vi "mean_2D.vi"(3 "transpose":bool, 4 "filter":enum16{"none", "invalids", "zero"}(ring), 5 "2D array":dbl[][](array[numeric])) -> (0 "errors":i32[](array[numeric]), 1 "counts":i32[](array[numeric]), 2 "means":dbl[](array[numeric]))   [LabVIEW 2020]
uses:
  <vilib>/Analysis/baseanly.llb/Mean (DBL).vi
  <vilib>/Analysis/NI_AALBase.lvlib
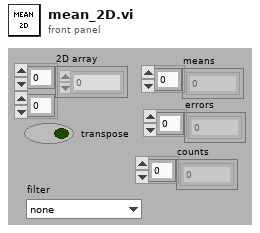
[diagram p1: front panel]
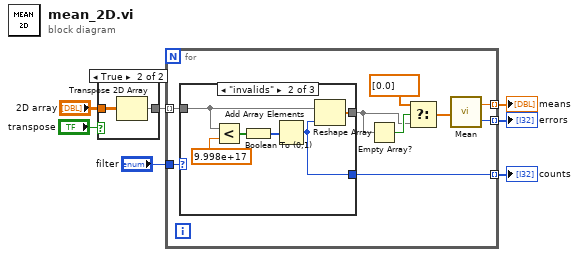
[diagram p0: block diagram]
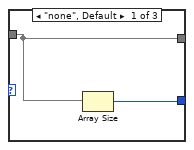
[diagram p3: hidden frame]
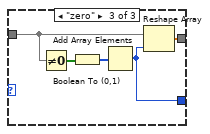
[diagram p4: hidden frame]
diagram:
  n1 = case shown="True" "transpose" {
    tunnel: "2D array" -> [w8 w10]
    tunnel: [w8 w9] -> w6
    frame False {
    }
    frame True {
      n2 = Transpose 2D Array(2D array=w10) -> (transposed array=w9:dbl[][])
    }
  }
  n3 = for {
    tunnel: w6 -> [w17] mode=indexing
    tunnel: [w19] -> w4 mode=indexing
    tunnel: [w18] -> w3 mode=indexing
    tunnel: [w16] -> w2 mode=indexing
    tunnel: "filter" -> [w15]
    n4 = case shown="\"invalids\"" w15 {
      tunnel: w17 -> [w21 w24 w28]
      tunnel: [w21 w23 w31] -> w12
      tunnel: [w20 w22 w30] -> w16
      frame "none", Default {
        n5 = Array Size(array=w21) -> (size(s)=w20:i32)
      }
      frame "invalids" {
        n6 = Less?(x=w24, y=9.998e+17) -> (x < y?=w26:bool[])
        n7 = Boolean To (0,1)(Boolean=w26) -> (0, 1=w25:i16[])
        n8 = Add Array Elements(numeric array=w25) -> (sum=w22:i16)
        n9 = Reshape Array(w24, w22) -> (w23:dbl[])
      }
      frame "zero" {
        n10 = Not Equal To 0?(x=w28) -> (x != 0?=w29:bool[])
        n11 = Boolean To (0,1)(Boolean=w29) -> (0, 1=w32:i16[])
        n12 = Add Array Elements(numeric array=w32) -> (sum=w30:i16)
        n13 = Reshape Array(w28, w30) -> (w31:dbl[])
      }
    }
    n14 = Empty Array?(array=w12) -> (empty?=w13:bool)
    n15 = Select(t=dbl[] [0.0], s=w13, f=w12) -> (s? t:f=w14:dbl[])
    n16 = call-poly <vilib>:"Mean.vi"("X"=w14) -> ("mean"=w19:dbl, "error"=w18:i32)
  }
  "means" <- w4
  "errors" <- w3
  "counts" <- w2
